vi "CalculateTimes.vi"(6 "Threshold (counts)":i32[](array[numeric])=[0, 0, 0, 0], 8 "error in":errorcluster, 9 "Dymin On?":bool, 10 "Laser Wait time (us)":dbl, 11 "DyMIN Step Times (us)":dbl[](array[numeric])=[0.0, 0.0, 0.0, 0.0] min=0.0 max=10000.0 step=0.0125) -> (0 "error out":errorcluster, 1 "PIX CLK period (bits)":i32, 2 "PIX CLK period (us)":dbl, 3 "All Step Times (bits)":i32[](array[numeric]), 4 "All Thresholds (counts)":i32[](array[numeric]), 5 "All Step Times (us)":dbl[](array[numeric]) min=0.0 max=1.0)   [LabVIEW 2016]
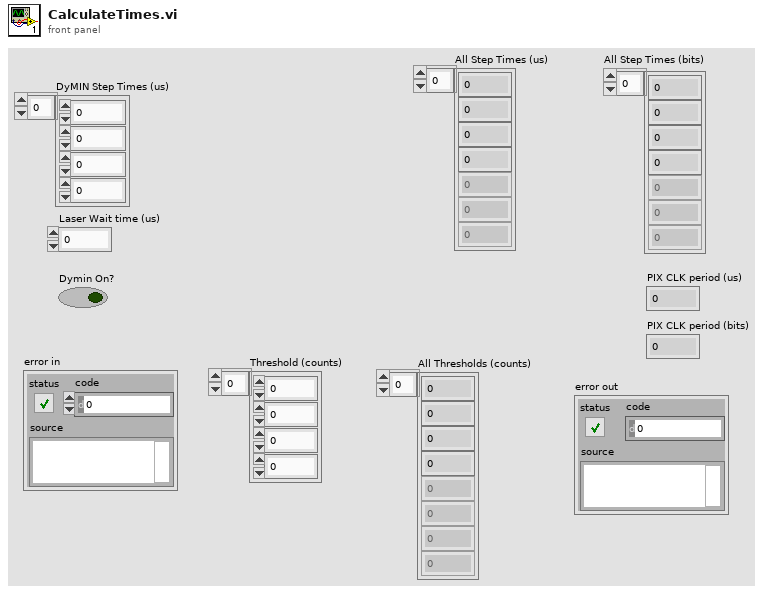
[diagram p1: front panel]
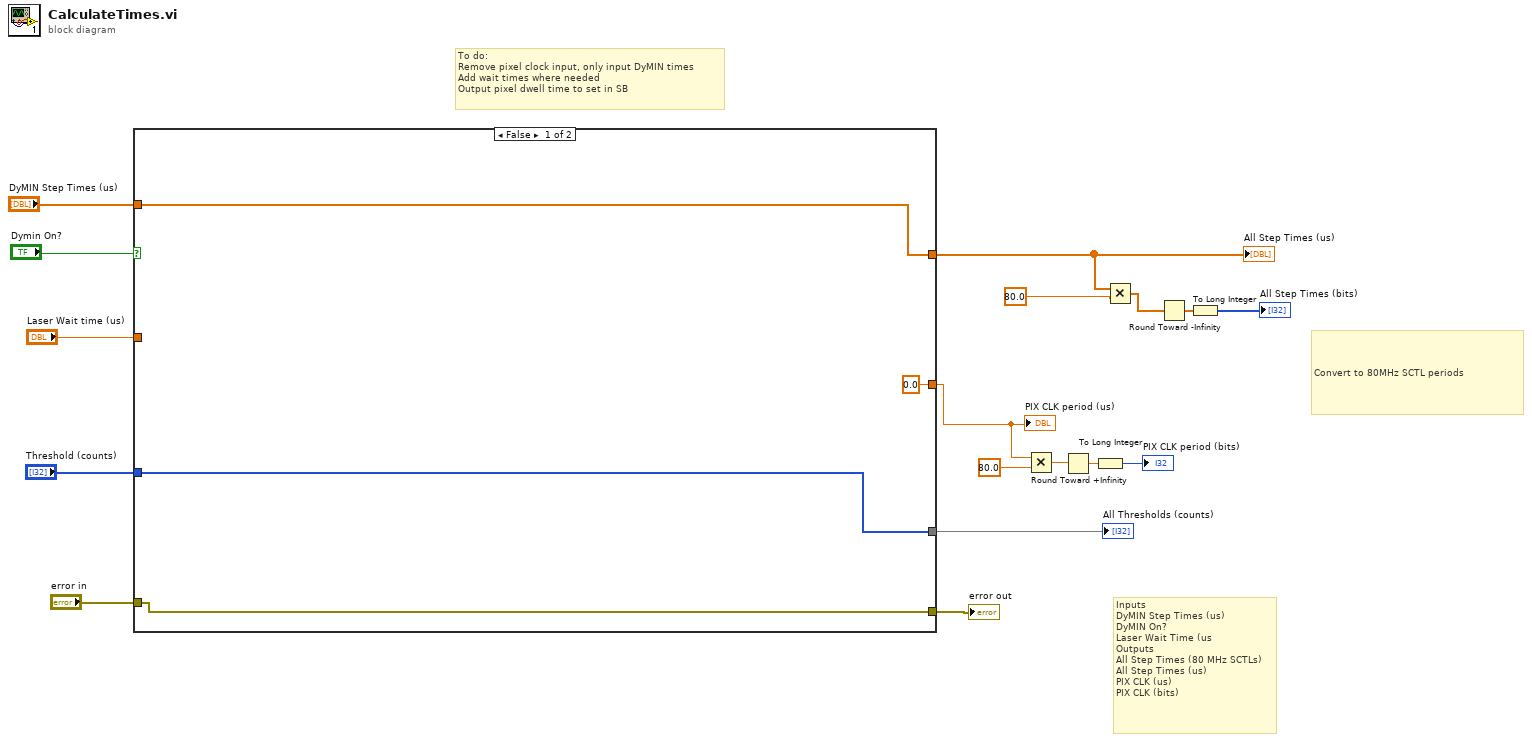
[diagram p0: block diagram]
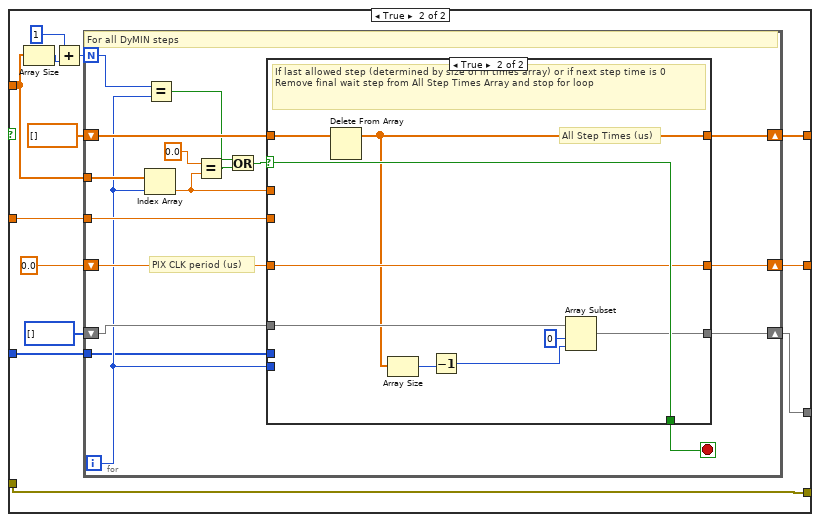
[diagram p2: hidden frame]
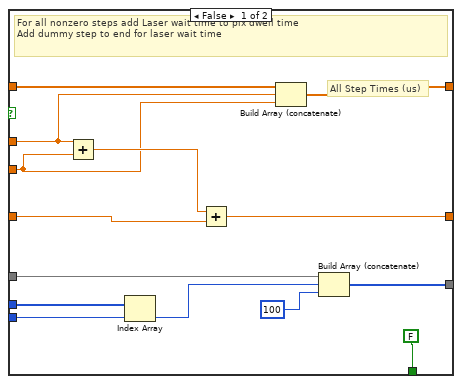
[diagram p3: hidden frame]
diagram:
  # "To do:\nRemove pixel clock input, only input DyMIN times\nAdd wait times where needed\nOutput pixel dwell time to set in SB"
  # "Inputs\nDyMIN Step Times (us)\nDyMIN On?\nLaser Wait Time (us\nOutputs\nAll Step Times (80 MHz SCTLs)\nAll Step Times (us)\nPIX CLK (us)\nPIX CLK (bits)"
  # "Convert to 80MHz SCTL periods"
  n1 = case shown="False" "Dymin On?" {
    tunnel: "DyMIN Step Times (us)" -> [w19 w31]
    tunnel: "error in" -> [w21 w30]
    tunnel: [w21 w30] -> w9
    tunnel: "Laser Wait time (us)" -> [_ w34]
    tunnel: [0.0 w29] -> w7
    tunnel: [w19 w28] -> w6
    tunnel: "Threshold (counts)" -> [w18 w25]
    tunnel: [w18 w22] -> w1
    frame False {
    }
    frame True {
      n2 = Array Size(array=w31) -> (size(s)=w23:i32)
      n3 = Add(x=1, y=w23) -> (x+y=w27:i32)
      n4 = for {
        N: w27 -> [w40]
        tunnel: w34 -> [w51]
        shift-right: [w41] -> w29
        shift-left: 0.0 -> [w50]
        shift-right: [w49] -> w28
        shift-left: dbl[] [] -> [w48]
        tunnel: w31 -> [w44]
        tunnel: w25 -> [w35]
        shift-right: [w38] -> w22
        shift-left: i32[] [] -> [w37]
        i -> [w36]
        stop <- w42 stop-if-true
        # "PIX CLK period (us)"
        # "For all DyMIN steps"
        n5 = Index Array(array=w44, index=w36) -> (element=w39:dbl)
        n6 = Equal?(x=w40, y=w36) -> (x = y?=w47:bool)
        n7 = Equal?(x=0.0 ("y"), y=w39) -> (x = y?=w46:bool)
        n8 = Or(x=w47, y=w46) -> (x .or. y?=w45:bool)
        n9 = case shown="True" w45 {
          selector: w45 -> [_ w73]
          tunnel: w51 -> [w63 _]
          tunnel: w50 -> [w65 w72]
          tunnel: [w62 w70] -> w49
          tunnel: w48 -> [w61 w74]
          tunnel: [FALSE w73] -> w42
          tunnel: [w59 w72] -> w41
          tunnel: w39 -> [w58 _]
          tunnel: [w57 w66] -> w38
          tunnel: w37 -> [w56 w71]
          tunnel: w36 -> [w55 _]
          tunnel: w35 -> [w52 _]
          frame False {
            # "All Step Times (us)"
            # "For all nonzero steps add Laser wait time to pix dwell time\nAdd dummy step to end for laser wait time"
            n10 = Add(x=w58, y=w63) -> (x+y=w64:dbl)
            n11 = Index Array(array=w52, index=w55) -> (element=w53:i32)
            n12 = Add(x=w64, y=w65) -> (x+y=w59:dbl)
            n13 = Build Array (concatenate)(w61, w58, w63) -> (w62:dbl[])
            n14 = Build Array (concatenate)(w56, w53, 100 ("element")) -> (w57:i32[])
          }
          frame True {
            # "All Step Times (us)"
            # "If last allowed step (determined by size of in times array) or if next step time is 0\nRemove final wait step from All Step Times Array and stop for loop"
            n15 = Delete From Array(array=w74) -> (array with subset deleted=w70:dbl[])  [unwired: 2 in, 1 out]
            n16 = Array Size(array=w70) -> (size(s)=w69:i32)
            n17 = Decrement(x=w69) -> (x-1=w67:i32)
            n18 = Array Subset(array=w71, index=0, length=w67) -> (w66:i32[])
          }
        }
      }
    }
  }
  "All Step Times (us)" <- w6
  "error out" <- w9
  "PIX CLK period (us)" <- w7
  "All Thresholds (counts)" <- w1
  n19 = Multiply(x=w7, y=80.0) -> (x*y=w14:dbl)
  n20 = Round Toward +Infinity(x=w14) -> (ceil(x): smallest int >= x=w13:dbl)
  n21 = To Long Integer(number=w13) -> (32bit integer=→"PIX CLK period (bits)":i32)
  n22 = Multiply(x=w6, y=80.0 ("element")) -> (x*y=w4:dbl[])
  n23 = Round Toward -Infinity(1:w4) -> (0:w17:dbl[])
  n24 = To Long Integer(number=w17) -> (32bit integer=→"All Step Times (bits)":i32[])
